vi "Link Channel Core.vi"(8 "error in (no error)":errorcluster, 10 "Channel Connection":T1, 11 "CIF_UI in":refnum<class "CIF_Manager_UI.lvclass">) -> (0 "error out":errorcluster, 3 "CIF_UI out":refnum<class "CIF_Manager_UI.lvclass">)   [LabVIEW 2021, in "CIF_Manager_UI.lvclass"]
uses:
  CIF_Manager_UI.lvclass
  C:/Program Files/National Instruments/LabVIEW 2021/vi.lib/CIF Foundation/CIF Core/CIFUI/CIF_UI.lvclass
  Typedef/Channel Connection.ctl
  <vilib>/CIF Foundation/CIF Core/CIFUI/CIF_UI.lvclass/CIF_UI.ctl
  <vilib>/CIF Foundation/CIF Core/CIFCore/Grpc/CIFCoreChannel_client/RPC Messages/cif_channelcore_SetConnectionRequest.ctl
  <vilib>/CIF Foundation/CIF Core/CIFCore/Grpc/CIFCoreChannel_client/RPC Messages/cif_management_common_ChannelPattern.ctl
  <vilib>/CIF Foundation/CIF Core/CIFCore/Common/Typedef/FIFO Publisher.ctl
  <vilib>/CIF Foundation/CIF Channels Core/ChannelCommon/typedef/New FIFO Instance Configuration.ctl
  <vilib>/CIF Foundation/CIF Core/CIFCore/Common/Typedef/Errors.ctl
  <vilib>/CIF Foundation/CIF Core/CIFUI/Accessors/Read Plugin Connection Map.vi
  <vilib>/CIF Foundation/CIF Core/CIFUI/Accessors/Read Channels.vi
  <vilib>/CIF Foundation/CIF Utilities/Errors/Append Error Location.vi
  <vilib>/CIF Foundation/CIF Core/CIFCore/Common/CIFCoreCommon.lvlib
  <vilib>/CIF Foundation/CIF Core/CIFCore/Grpc/CIFCoreWrapper/CIFCoreWrapper.lvlib
  <vilib>/CIF Foundation/CIF Core/CIFCore/Grpc/CIFCoreChannel_client/CIFCoreChannel_client.lvlib
  <vilib>/CIF Foundation/CIF Channels Core/ChannelCommon/ChannelCommon.lvlib
  <vilib>/CIF Foundation/CIF Core/CIFUI/CIF_UI.lvclass
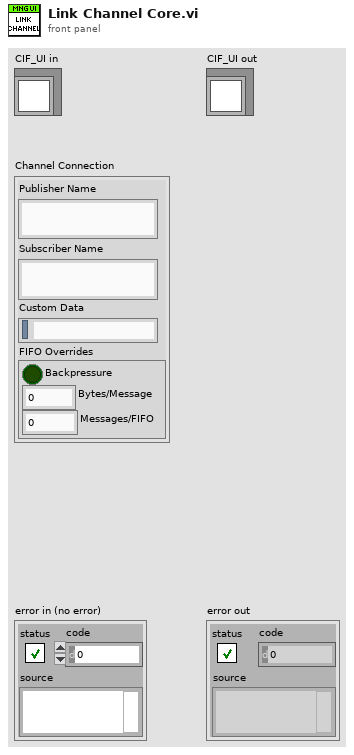
[diagram p1: front panel]
types:
  T1 = typedef "CIF_Manager_UI.lvclass/Channel Connection.ctl" = cluster{"Publisher Name":string, "Subscriber Name":string, "Custom Data":string, "FIFO Overrides":cluster{"Backpressure":bool, "Bytes/Message":u32, "Messages/FIFO":u32}}
  T2 = typedef "CIFCoreChannel_client.lvlib/cif_channelcore_SetConnectionRequest.ctl" = cluster{"subscriber_name":string, "publisher_name":string, "custom_connect":u8[]}
  T3 = typedef "CIFCoreChannel_client.lvlib/cif_management_common_Channel.ctl" = cluster{"name":string, "direction":T4, "type":string, "custom_config":u8[], "connected":bool, "connected_name":string, "forced":bool, "channel_pattern":T5}
  T4 = typedef "CIFCoreChannel_client.lvlib/cif_management_common_ChannelDirection.ctl" = enum32{"CHANNELDIRECTION_UNKNOWN", "CHANNELDIRECTION_PUBLISHER", "CHANNELDIRECTION_SUBSCRIBER"}
  T5 = typedef "CIFCoreChannel_client.lvlib/cif_management_common_ChannelPattern.ctl" = enum32{"CHANNELPATTERN_UNKNOWN", "CHANNELPATTERN_TAG", "CHANNELPATTERN_FIFO", "CHANNELPATTERN_MULTIFIFO", "CHANNELPATTERN_BACKPRESSUREFIFO"}
  T6 = typedef "CIFCoreCommon.lvlib/FIFO Publisher.ctl" = cluster{"Publisher Name":string, "New FIFO Instance Config":T7}
  T7 = typedef "ChannelCommon.lvlib/New FIFO Instance Configuration.ctl" = cluster{"Backpressure":bool, "Bytes/Message Override":u32, "Messages/FIFO Override":u32, "Custom Data":u8[]}
  T8 = typedef "CIFCoreCommon.lvlib/Errors.ctl" = enum16{"Invalid Clock ID", "Long Sleep", "gRPC Server Not Found", "Config Parse", "Timestamp Wrap", "Delayed Execution", "Duplicate Channel", "Missing Channel", "Incorrect Type", "Flatten Error", "Unflatten Data", "Unique Name", "Plugin Not Found", "Plugin Type Not Found", "Plugin Version Not Found", "Manager Not Found", "Numerical Issue", "Time Jump", "Clock ID Match", "Channel Length", "Plugin Connection", "gRPC Server Connection", "PPL Name Match", "Build", "Config Log Parse", "Plugin Load", "UI Subpanel Load", "Python Name", "Invalid Name", "Unable to Change Ch Buffer", "Failed Kill", "Failed SysExec", "Function Not Implemented", "Load Timeout"}
  T9 = typedef "CIF_UI.lvclass/Plugin Connection Map.ctl" = map{string, T10}
  T10 = typedef "CIF_UI.lvclass/Plugin Connections.ctl" = cluster{"gRPC ID":T11, "Plugin Info":T12}
  T11 = typedef "grpc-lvsupport-release.lvlib/grpcId.ctl" = u64
  T12 = typedef "CIFCoreCommon.lvlib/PluginInfo.ctl" = cluster{"Name":string, "Type":string, "grpc_port":i32, "Version":T13, "Node Status":T14}
  T13 = typedef "CIFCoreCommon.lvlib/Version Simple.ctl" = cluster{"Major":i32, "Minor":i32, "Fix":i32}
  T14 = typedef "CIFCoreCommon.lvlib/gRPC Reported Plugin Status.ctl" = cluster{"State":T15, "Timing Statistics (us)":T16, "FIFO Statistics (us)":T18, "error":T19, "Monitor Doubles":T20, "Monitor U64":T21, "Monitor I64":T22}
  T15 = typedef "CIFCoreCommon.lvlib/Plugin State.ctl" = enum32{"Null", "Creating", "Listening", "Running", "CleaningUp", "Destroying"}
  T16 = typedef "CIFCoreCommon.lvlib/Timing Statistics.ctl" = cluster{"Period":T17, "Wake Error":T17, "Execute":T17, "Housekeep":T17, "Idle":T17, "Cleanup":T17, "Custom 1 (custom units)":T17, "Custom 2 (custom units)":T17}
  T17 = typedef "CIFCoreCommon.lvlib/Timing Stats Base.ctl" = cluster{"Max":i64, "Avg":dbl, "Min":i64}
  T18 = typedef "CIFCoreCommon.lvlib/FIFO Statistics.ctl" = cluster{"From T0":T17, "From Previous Plugin":T17, "Output Error":T17}
  T19 = typedef "CIFCoreCommon.lvlib/Simple Error.ctl" = cluster{"status":bool, "code":i32}
  T20 = typedef "CIFCoreCommon.lvlib/Monitor Doubles.ctl" = cluster{"1":dbl, "2":dbl, "3":dbl, "4":dbl}
  T21 = typedef "CIFCoreCommon.lvlib/Monitor U64.ctl" = cluster{"1":u64, "2":u64, "3":u64, "4":u64}
  T22 = typedef "CIFCoreCommon.lvlib/Monitor I64.ctl" = cluster{"1":i64, "2":i64, "3":i64, "4":i64}
  T23 = typedef "ChannelCommon.lvlib/New FIFO Instance Response.ctl" = cluster{"Publisher":string, "Custom Data":u8[]}
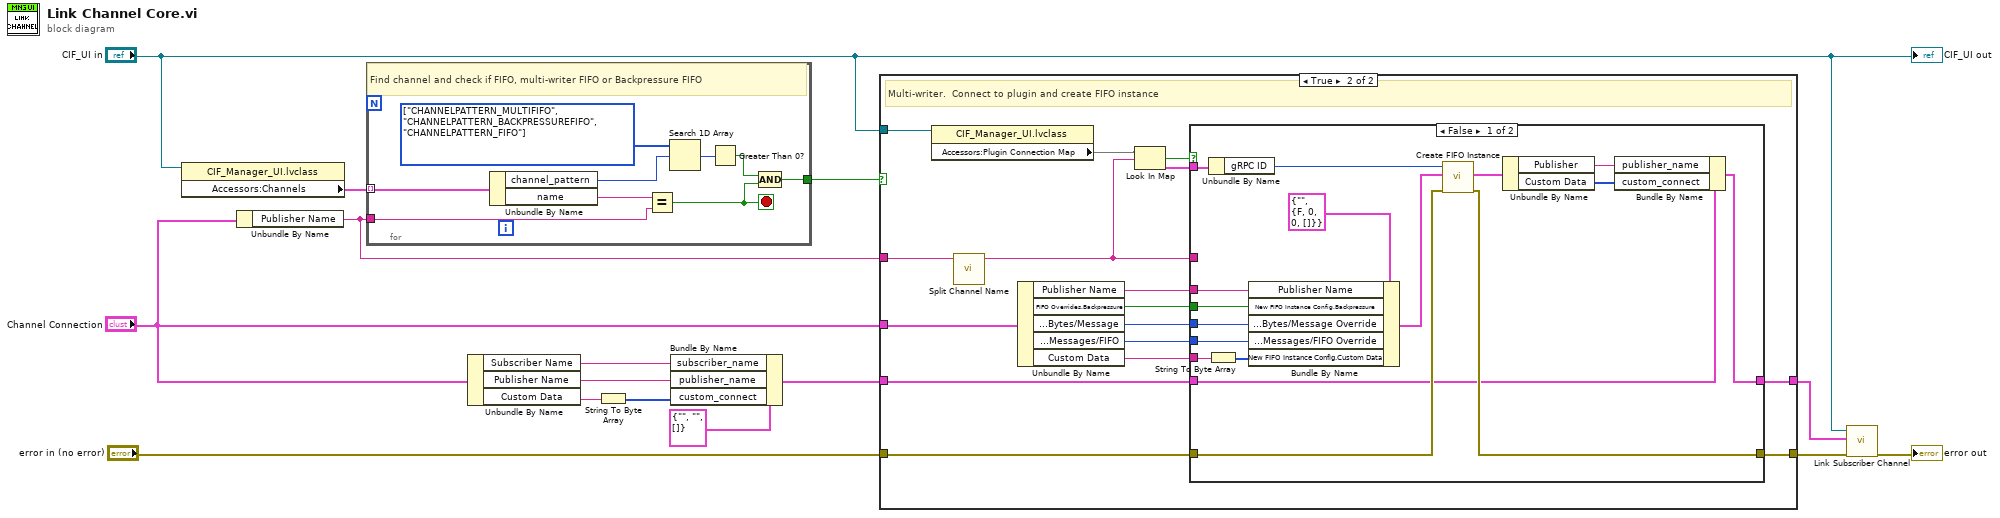
[diagram p0: block diagram]
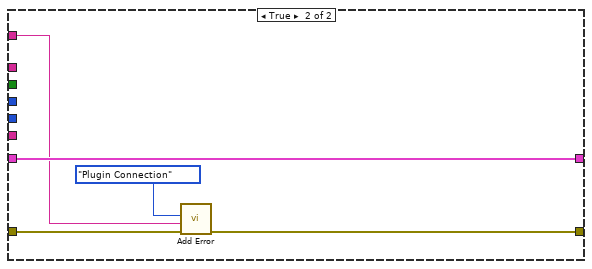
[diagram p3: hidden frame]
diagram:
  n1 = property class="CIF_Manager_UI.lvclass"(reference="CIF_UI in") -> ("Accessors:Channels"=w1:T3[])  [unwired: 1 in, 2 out]
  n2 = Unbundle By Name("Channel Connection") -> ("Publisher Name"=w15:string)
  n3 = for {
    tunnel: w1 -> [w24] mode=indexing
    tunnel: [w21] -> w14
    tunnel: w15 -> [w20]
    stop <- w22 stop-if-true
    w19 = T5[] [enum."CHANNELPATTERN_MULTIFIFO", enum."CHANNELPATTERN_BACKPRESSUREFIFO", enum."CHANNELPATTERN_FIFO"] items=["CHANNELPATTERN_UNKNOWN", "CHANNELPATTERN_TAG", "CHANNELPATTERN_FIFO", "CHANNELPATTERN_MULTIFIFO", "CHANNELPATTERN_BACKPRESSUREFIFO"] ("1D array")
    # "Find channel and check if FIFO, multi-writer FIFO or Backpressure FIFO"
    n4 = Unbundle By Name(w24) -> ("channel_pattern"=w18:T5, "name"=w23:string)
    n5 = Equal?(x=w23, y=w20) -> (x = y?=w22:bool)
    n6 = Search 1D Array(1D array=w19, element=w18) -> (index of element=w17:i32)  [unwired: 1 in]
    n7 = Greater Than 0?(x=w17) -> (x > 0?=w16:bool)
    n8 = Compound Arithmetic op=AND(w16, w22) -> (w21:bool)
  }
  n9 = Unbundle By Name("Channel Connection") -> ("Subscriber Name"=w10:string, "Publisher Name"=w9:string, "Custom Data"=w8:string)
  n10 = String To Byte Array(string=w8) -> (unsigned byte array=w12:u8[])
  n11 = Bundle By Name(cluster=T2 {"subscriber_name"="", "publisher_name"="", "custom_connect"=[]} ("Connection"), "subscriber_name"=w10, "publisher_name"=w9, "custom_connect"=w12) -> (w7:T2)
  n12 = case shown="True" w14 {
    tunnel: w15 -> [_ w31]
    tunnel: "CIF_UI in" -> [_ w28]
    tunnel: "error in (no error)" -> [w25 w40]
    tunnel: "Channel Connection" -> [_ w39]
    tunnel: w7 -> [w26 w34]
    tunnel: [w26 w33] -> w5
    tunnel: [w25 w32] -> w6
    frame False {
      # "Not a multi-writer FIFO.  No need to contact publisher."
    }
    frame True {
      # "Multi-writer.  Connect to plugin and create FIFO instance"
      n13 = property class="CIF_Manager_UI.lvclass"(reference=w28) -> ("Accessors:Plugin Connection Map"=w27:T9)  [unwired: 1 in, 2 out]
      n14 = call <vilib>:"Split Channel Name.vi"("Channel Name"=w31) -> ("Parent"=w30:string)  [unwired: 8 in, 2 out]
      n15 = Unbundle By Name(w39) -> ("Publisher Name"=w38:string, "FIFO Overrides.Backpressure"=w37:bool, "FIFO Overrides.Bytes/Message"=w36:u32, "FIFO Overrides.Messages/FIFO"=w35:u32, "Custom Data"=w29:string)
      n16 = Look In Map(map=w27, key=w30) -> (key not found?=w42:bool, value=w41:T10)  [unwired: 1 in]
      n17 = case shown="False" w42 {
        tunnel: w41 -> [w59 _]
        tunnel: [w58 w62] -> w32
        tunnel: w40 -> [w56 w63]
        tunnel: w30 -> [_ w61]
        tunnel: w38 -> [w55 _]
        tunnel: w37 -> [w54 _]
        tunnel: w36 -> [w53 _]
        tunnel: w35 -> [w52 _]
        tunnel: w34 -> [w51 w64]
        tunnel: [w50 w64] -> w33
        tunnel: w29 -> [w44 _]
        frame False {
          n18 = String To Byte Array(string=w44) -> (unsigned byte array=w43:u8[])
          n19 = Unbundle By Name(w59) -> ("gRPC ID"=w57:T11)
          n20 = Bundle By Name(cluster=T6 {"Publisher Name"="", "New FIFO Instance Config"={"Backpressure"=FALSE, "Bytes/Message Override"=0, "Messages/FIFO Override"=0, "Custom Data"=[]}} ("New Publisher"), "Publisher Name"=w55, "New FIFO Instance Config.Backpressure"=w54, "New FIFO Instance Config.Bytes/Message Override"=w53, "New FIFO Instance Config.Messages/FIFO Override"=w52, "New FIFO Instance Config.Custom Data"=w43) -> (w48:T6)
          n21 = call <vilib>:"Create FIFO Instance.vi"("error in"=w56, "New Publisher"=w48, "gRPC ID"=w57) -> ("error out"=w58:errorcluster, "FIFO Instance"=w47:T23)  [unwired: 6 in, 1 out]
          n22 = Unbundle By Name(w47) -> ("Publisher"=w46:string, "Custom Data"=w45:u8[])
          n23 = Bundle By Name(cluster=w51, "publisher_name"=w46, "custom_connect"=w45) -> (w50:T2)
        }
        frame True {
          n24 = call <vilib>:"Add Error.vi"("error in (no error)"=w63, "String to Append"=w61, "Error"=Errors."Plugin Connection") -> ("error out"=w62:errorcluster)  [unwired: 8 in]
        }
      }
    }
  }
  n25 = call <vilib>:"Link Subscriber Channel.vi"("error in (no error)"=w6, "Connection"=w5, "CIF_UI in"="CIF_UI in") -> ("error out"=→"error out":errorcluster)  [unwired: 8 in]
  "CIF_UI out" <- "CIF_UI in"
